vi "top2.vi"() -> ()   [LabVIEW 2014]
panel:
  out "Waveform Chart 2":T1(graph)
  in  "Celsius / Fahrenheit":bool
  in  "summer / winter":bool
  in  "summer upper bound":dbl
  in  "summer lower bound":dbl
  in  "winter upper bound":dbl
  in  "winter lower bound":dbl
  in  "stop":bool
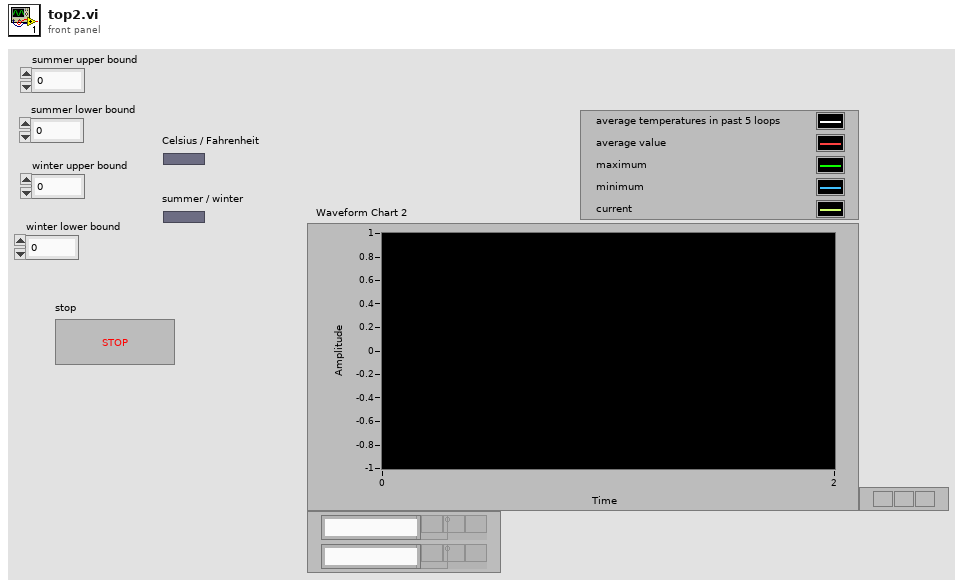
[diagram p1: front panel]
types:
  T1 = cluster{dbl, dbl, "Deg C":dbl, "Deg C":dbl, "Deg C":dbl}
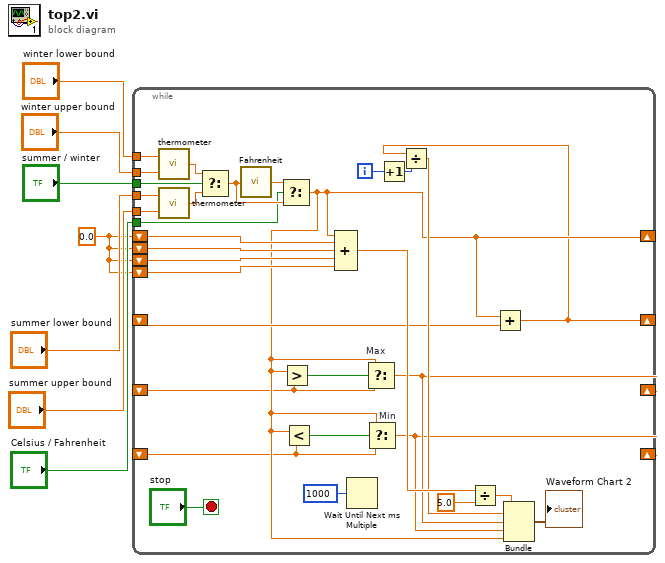
[diagram p0: block diagram]
diagram:
  w1 = 0.0 ("Deg C")
  n1 = while {
    tunnel: "winter lower bound" -> [w34]
    tunnel: "winter upper bound" -> [w33]
    tunnel: "summer lower bound" -> [w32]
    tunnel: "summer upper bound" -> [w31]
    tunnel: "Celsius / Fahrenheit" -> [w30]
    tunnel: "summer / winter" -> [w29]
    shift-right: [w15] -> _
    shift-left: w1 -> [w25]
    shift-left: w1 -> [w19]
    shift-left: w1 -> [w18]
    shift-left: w1 -> [w17]
    shift-right: [w14] -> _
    shift-left: _ -> [w16]
    shift-right: [w13] -> _
    shift-left: _ -> [w11]
    shift-right: [w12] -> _
    shift-left: _ -> [w10]
    i -> [w28]
    stop <- "stop" stop-if-true
    n2 = call "thermometer.vi"("upper bound"=w33, "lower bound"=w34) -> ("Deg C"=w37:dbl)
    n3 = call "thermometer.vi"("upper bound"=w31, "lower bound"=w32) -> ("Deg C"=w36:dbl)
    n4 = Select(t=w37, s=w29, f=w36) -> (s? t:f=w39:dbl)
    n5 = call "Fahrenheit.vi"("Deg C"=w39) -> ("Deg F"=w38:dbl)
    n6 = Select(t=w38, s=w30, f=w39) -> (s? t:f=w15:dbl)
    n7 = Greater?(x=w15, y=w11) -> (0:w27:bool)
    n8 = Less?(x=w15, y=w10) -> (x < y?=w26:bool)
    n9 = Compound Arithmetic op=ADD(w15, w25, w19, w18, w17) -> (w22:dbl)
    n10 = Wait Until Next ms Multiple(millisecond multiple=u32 1000) -> ()  [unwired: 1 out]
    n11 = Select "Max"(t=w15, s=w27, f=w11) -> (s? t:f=w13:dbl)
    n12 = Select "Min"(t=w15, s=w26, f=w10) -> (s? t:f=w12:dbl)
    n13 = Increment(x=w28) -> (x+1=w20:i32)
    n14 = Divide(x=w22, y=5.0) -> (x/y=w24:dbl)
    n15 = Add(x=w15, y=w16) -> (x+y=w14:dbl)
    n16 = Divide(x=w14, y=w20) -> (x/y=w21:dbl)
    n17 = Bundle(w24, w21, "Deg C"=w13, "Deg C"=w12, "Deg C"=w15) -> (→"Waveform Chart 2":T1)  [unwired: 1 in]
  }
